vi "Last Ack Created.vi"(7 "Sender":refnum<class "Sender.lvclass">, 10 "jettl":refnum<class "jettl.lvclass">, 11 "Last Ack Created in":refnum<class "Last Ack Created.lvclass">) -> (3 "Last Ack Created out":refnum<class "Last Ack Created.lvclass">)   [LabVIEW 2021, in "jettl.lvlib" / "Last Ack Created Msg Strategy.lvlib" / "Last Ack Created.lvclass"]
uses:
  Last Ack Created.lvclass
  jettl/jettl.lvclass
  Sender/Sender/Sender.lvclass
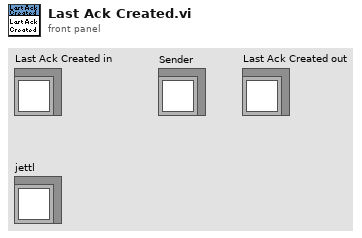
[diagram p1: front panel]
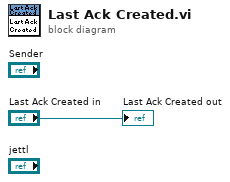
[diagram p0: block diagram]
diagram:
  "Last Ack Created out" <- "Last Ack Created in"
